vi "Real Matrix Logarithm_Check Normal.vi"(9 "tolerance":dbl, 10 "Eigenvalues":cdb[](array[numeric]), 11 "Schur Form":T1) -> (3 "normal?":bool)   [LabVIEW 2010, in "NI_AALBase.lvlib"]
uses:
  NI_AALBase.lvlib
  RealMatrix.ctl
  NI_Matrix.lvlib
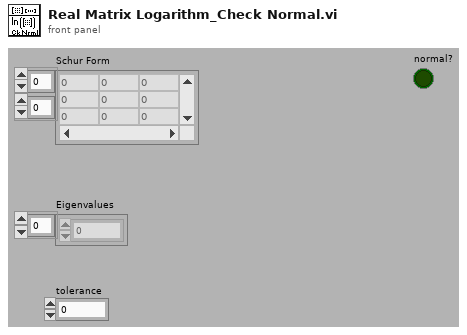
[diagram p1: front panel]
types:
  T1 = typedef "NI_Matrix.lvlib/RealMatrix.ctl" = dbl[][]
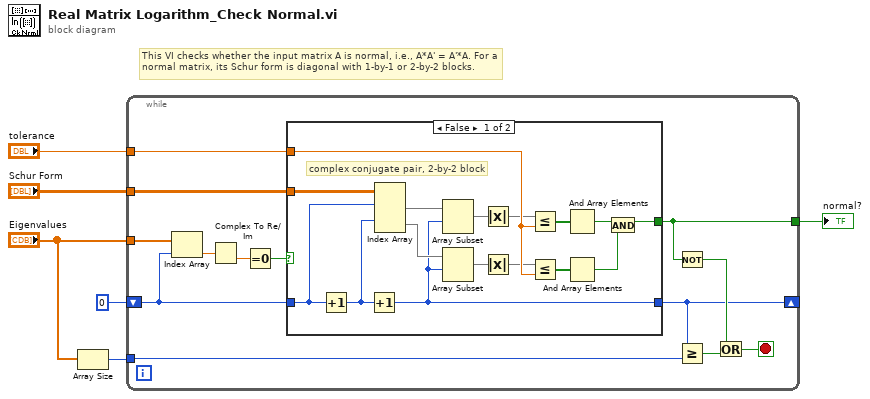
[diagram p0: block diagram]
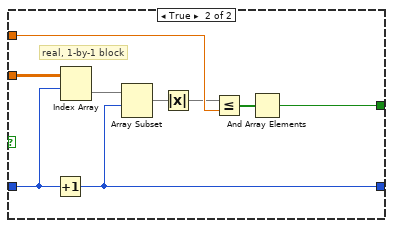
[diagram p2: hidden frame]
diagram:
  # "This VI checks whether the input matrix A is normal, i.e., A*A' = A'*A. For a normal matrix, its Schur form is diagonal with 1-by-1 or 2-by-2 blocks."
  n1 = Array Size(array="Eigenvalues") -> (size(s)=w5:i32)
  n2 = while {
    tunnel: "Eigenvalues" -> [w19]
    tunnel: w5 -> [w15]
    tunnel: "Schur Form" -> [w14]
    tunnel: "tolerance" -> [w13]
    tunnel: [w9] -> w1
    shift-right: [w8] -> _
    shift-left: 0 -> [w7]
    stop <- w10 stop-if-true
    n3 = Index Array(array=w19, index=w7) -> (element=w18:cdb)
    n4 = Complex To Re/Im(x + iy=w18) -> (y=w17:dbl)  [unwired: 1 out]
    n5 = Equal To 0?(x=w17) -> (x = 0?=w16:bool)
    n6 = case shown="False" w16 {
      tunnel: w7 -> [w34 w43]
      tunnel: [w30 w41] -> w8
      tunnel: w14 -> [w35 w44]
      tunnel: w13 -> [w26 w40]
      tunnel: [w22 w37] -> w9
      frame False {
        # "complex conjugate pair, 2-by-2 block"
        n7 = Increment(x=w34) -> (x+1=w33:i32)
        n8 = Increment(x=w33) -> (x+1=w30:i32)
        n9 = Index Array(array=w35, index (row) #1=w34, index (row) #2=w33) -> (element #1=w32:dbl[], element #2=w31:dbl[])  [unwired: 2 in]
        n10 = Array Subset(array=w32, index=w30) -> (w28:dbl[])  [unwired: 1 in]
        n11 = Array Subset(array=w31, index=w30) -> (w25:dbl[])  [unwired: 1 in]
        n12 = Absolute Value(x=w28) -> (abs(x)=w21:dbl[])
        n13 = Absolute Value(x=w25) -> (abs(x)=w20:dbl[])
        n14 = Less Or Equal?(x=w21, y=w26) -> (x <= y?=w29:bool[])
        n15 = Less Or Equal?(x=w20, y=w26) -> (x <= y?=w27:bool[])
        n16 = And Array Elements(Boolean array=w29) -> (logical AND=w24:bool)
        n17 = And Array Elements(Boolean array=w27) -> (logical AND=w23:bool)
        n18 = And(x=w24, y=w23) -> (x .and. y?=w22:bool)
      }
      frame True {
        # "real, 1-by-1 block"
        n19 = Increment(x=w43) -> (x+1=w41:i32)
        n20 = Index Array(array=w44, index (row)=w43) -> (element=w42:dbl[])  [unwired: 1 in]
        n21 = Array Subset(array=w42, index=w41) -> (w39:dbl[])  [unwired: 1 in]
        n22 = Absolute Value(x=w39) -> (abs(x)=w36:dbl[])
        n23 = Less Or Equal?(x=w36, y=w40) -> (x <= y?=w38:bool[])
        n24 = And Array Elements(Boolean array=w38) -> (logical AND=w37:bool)
      }
    }
    n25 = Not(x=w9) -> (.not. x?=w12:bool)
    n26 = Greater Or Equal?(x=w8, y=w15) -> (x >= y?=w11:bool)
    n27 = Or(x=w12, y=w11) -> (x .or. y?=w10:bool)
  }
  "normal?" <- w1
